vi "flash_RPCV2.vi"() -> ()   [LabVIEW 2017]
panel:
  out "error out 2":errorcluster
  out "Out 2":u8=4 format="%.0x"
  in  "Firmware":u16(ring)=4 items=["SP6"=4, "Middle"=3, "Final"=2]
  out "Out":u8 format="%.0x"
  out "字符串 2":string
  out "concatenated string":string
  in  "Register_Base_Address":u32=512 format="%x"
  in  "start":bool=TRUE
  out "Current IP address":string="192.168.10.20"
  in  "IP address list":string[](array[string])=["192.168.10.20"]
  in  "回读":bool
  out "Current Progress":u32(slide)=342016 scale=0.0..341712.0
  out "error out":errorcluster={"status"=TRUE, "code"=4, "source"="Read from Binary File in flash_RPCV1.vi<APPEND>\nG:\\rpc\\FPGA\\top.bin"}
  out "appended array":bool[](array[boolean])
  out "Process":u32=342016
  in  "error in (no error)":errorcluster
  in  "Read (TRUE)":bool
  out "byte data":string
  out "Total size (in bytes)":i64=341988
  in  "file path (use dialog)":path=path "G:/rpc/FPGA/top_sp6.bin"
  # "FF80 0001 0000 0209 13"
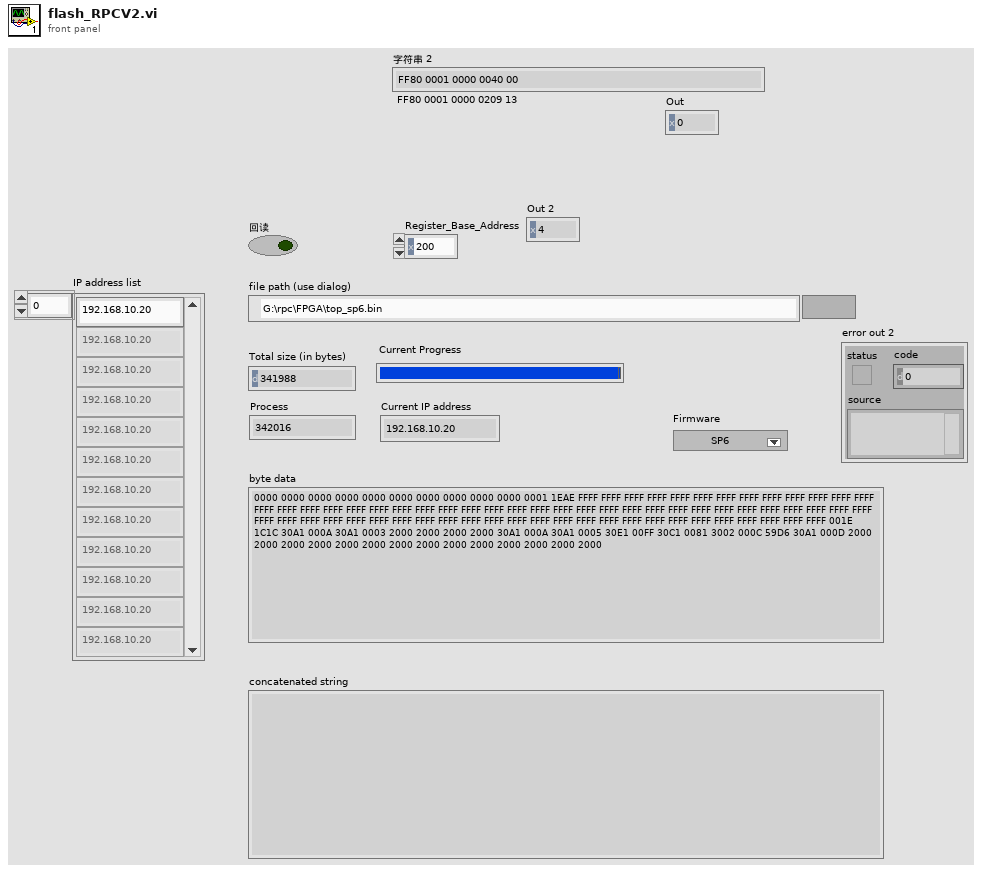
[diagram p1: front panel]
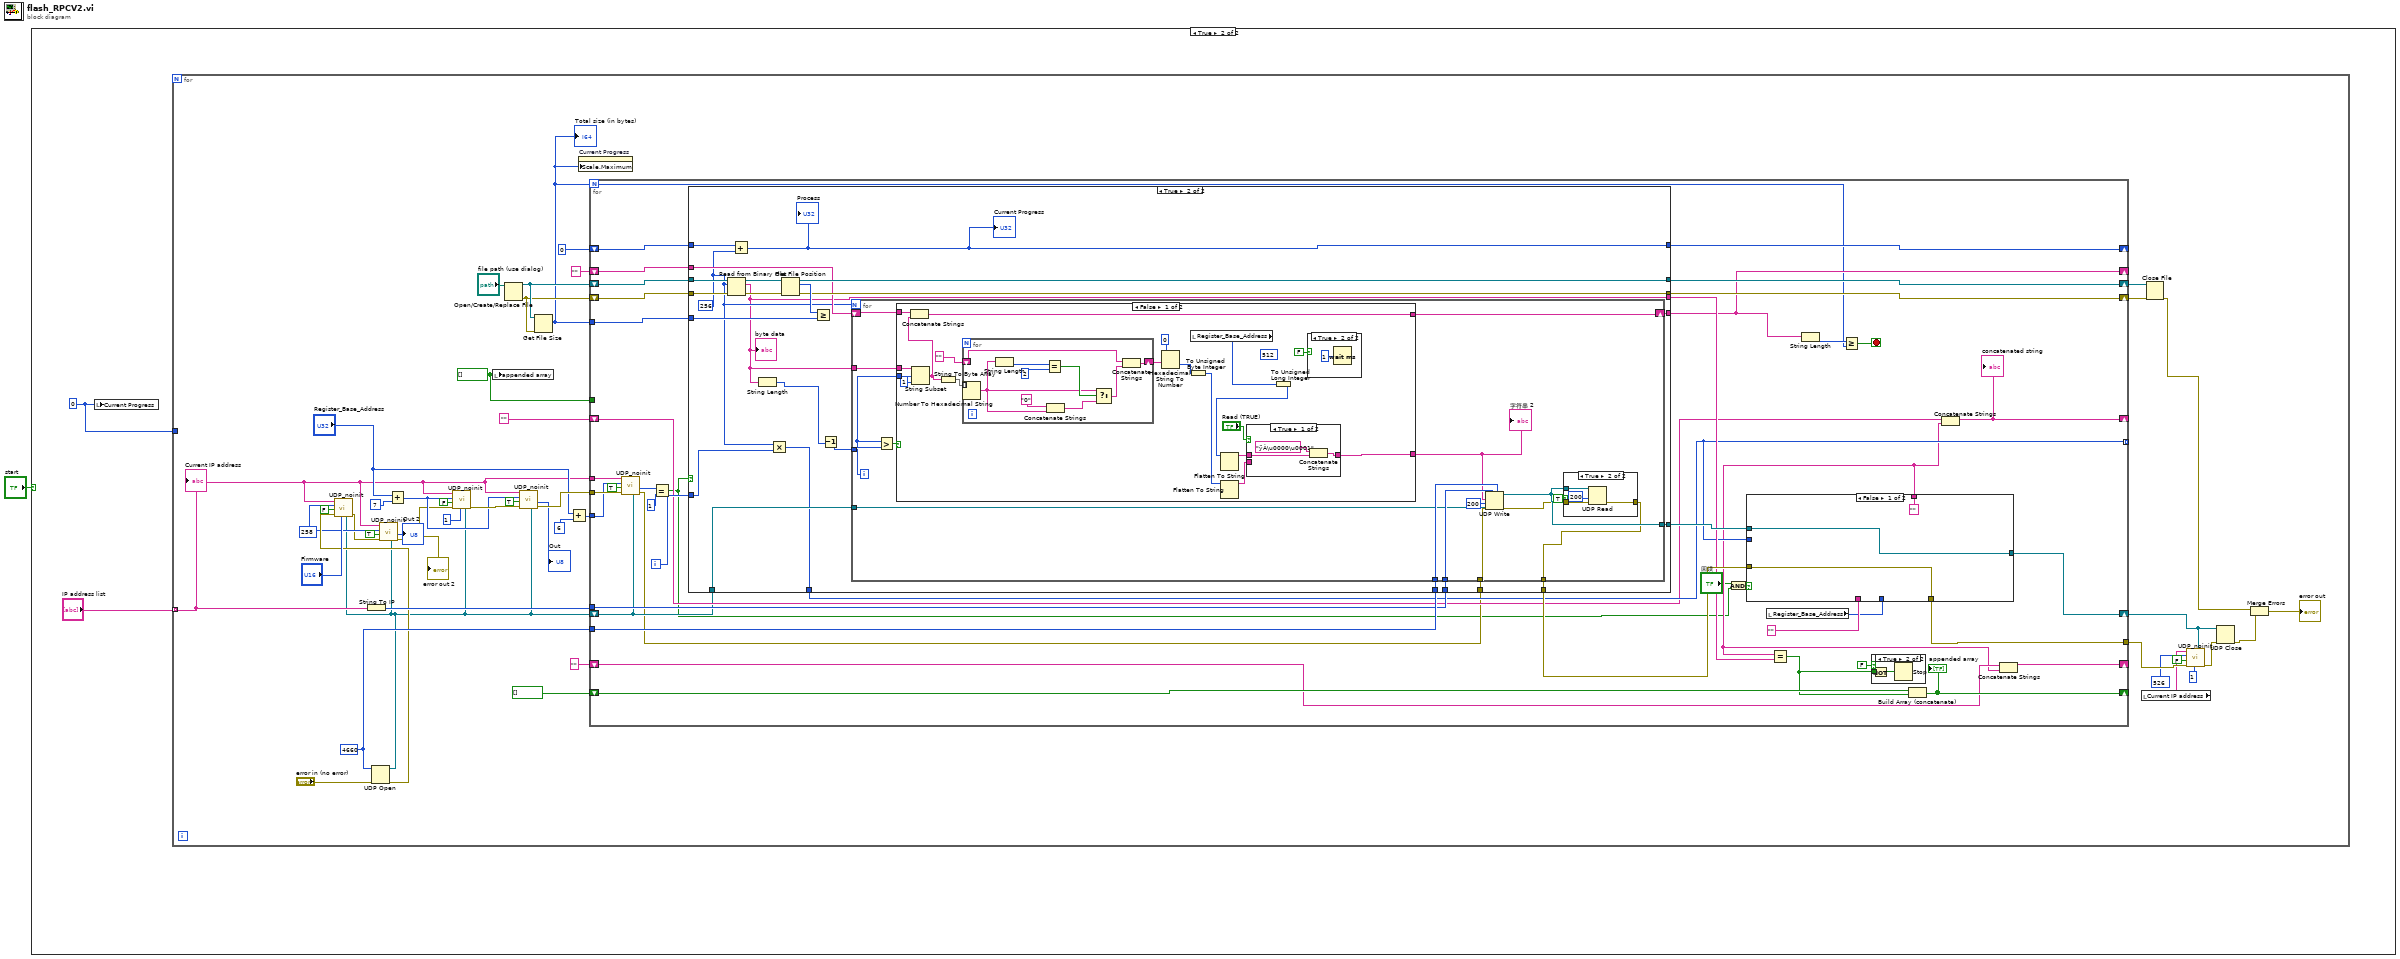
[diagram p0: block diagram]
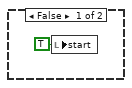
[diagram p2: hidden frame]
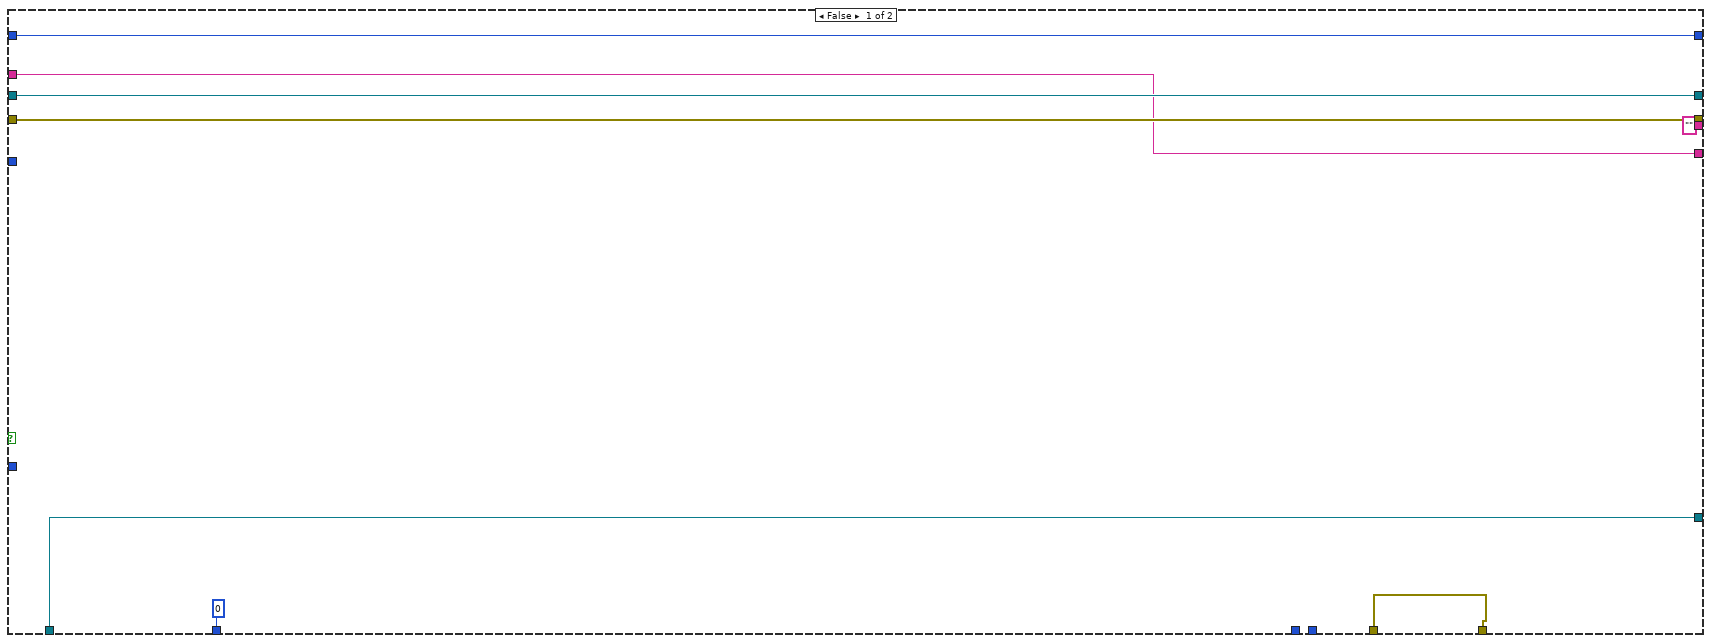
[diagram p3: hidden frame]
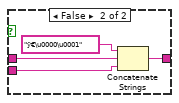
[diagram p5: hidden frame]
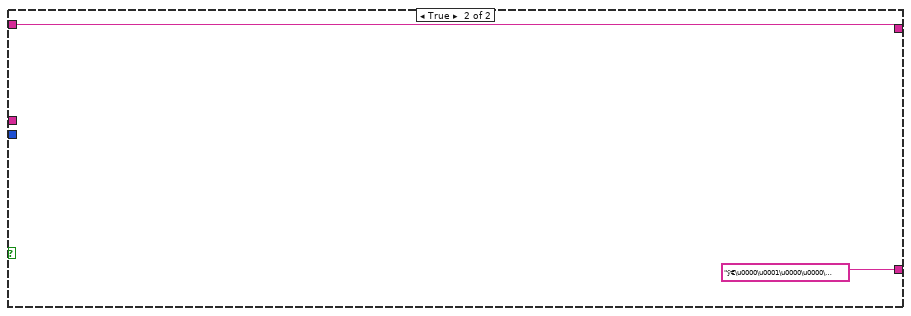
[diagram p7: hidden frame]
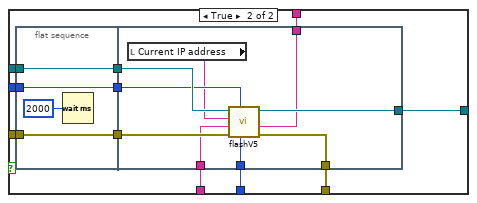
[diagram p8: hidden frame]
diagram:
  n1 = case shown="True" "start" {
    frame False {
      n2 = local write "start"(TRUE ("start")) -> ()
    }
    frame True {
      w3 = u8 0 ("In")
      n3 = local write "Current Progress"(w3) -> ()
      n4 = for {
        tunnel: "IP address list" -> [w18] mode=indexing
        tunnel: w3 -> [_]
        w17 = u32 258 ("Address")
        w32 = bool[] [] ("appended array")
        w45 = u16 4660 ("UDP port")
        n5 = String To IP(1:w18) -> (0:w44:u32)
        n6 = UDP Open(8:"error in (no error)", 11:w45) -> (port=w14:refnum<k16>, 0:w19:errorcluster)  [unwired: 3 in, 1 out]
        n7 = call "UDP_noinit.vi"("connection ID"=w14, "In"="Firmware", "error in (no error)"=w19, "Read (TRUE)"=FALSE, "Address"=w17, "IP address"=w18) -> ("error out"=w13:errorcluster)  [unwired: 2 in, 2 out]
        n8 = call "UDP_noinit.vi"("connection ID"=w14, "error in (no error)"=w13, "Read (TRUE)"=TRUE, "Address"=w17, "IP address"=w18) -> ("error out"=w12:errorcluster, "Out"=→"Out 2":u8)  [unwired: 3 in, 1 out]
        "error out 2" <- w12
        n9 = Add(x="Register_Base_Address", y=u32 7 ("Address")) -> (x+y=w27:u32)
        n10 = call "UDP_noinit.vi"("connection ID"=w14, "In"=u8 1, "error in (no error)"=w12, "Read (TRUE)"=FALSE, "Address"=w27, "IP address"=w18) -> ("error out"=w36:errorcluster)  [unwired: 2 in, 2 out]
        n11 = local write "appended array"(w32) -> ()
        n12 = Open/Create/Replace File(file path (use dialog)="file path (use dialog)") -> (refnum out=w49:refnum<file>, error out=w48:errorcluster)  [unwired: 5 in, 1 out]
        n13 = call "UDP_noinit.vi"("connection ID"=w14, "error in (no error)"=w36, "Read (TRUE)"=TRUE, "Address"=w27, "IP address"=w18) -> ("error out"=w38:errorcluster, "Out"=→"Out":u8)  [unwired: 3 in, 1 out]
        n14 = Get File Size(file=w49, error in=w48) -> (size (in bytes)=w33:i64)  [unwired: 2 out]
        "Total size (in bytes)" <- w33
        n15 = Add(x="Register_Base_Address", y=u32 6 ("Address")) -> (x+y=w24:u32)
        n16 = property on="Current Progress" class="Slide (strict)"("Scale.Maximum"=w33) -> ()  [unwired: 2 in, 2 out]
        n17 = for {
          N: w33 -> [w70]
          tunnel: w33 -> [w91]
          shift-right: [w90] -> w47
          shift-left: w48 -> [w92]
          shift-right: [w89] -> w46
          shift-left: w49 -> [w93]
          shift-right: [w72] -> _
          shift-left: "" -> [w88]
          tunnel: w45 -> [w85]
          tunnel: [w80] -> w10
          tunnel: w44 -> [w84]
          shift-right: [w82] -> w6
          shift-left: w14 -> [w60]
          shift-right: [w86] -> _
          shift-left: u32 0 ("length (rest)") -> [w87]
          shift-right: [w77] -> _
          shift-left: bool[] [] -> [w75]
          tunnel: [w73] -> _ mode=indexing
          shift-right: [w68] -> _
          shift-left: "" -> [w67]
          tunnel: w18 -> [w65]
          tunnel: w38 -> [w59]
          shift-right: [w57] -> _
          shift-left: "" -> [w56]
          tunnel: w32 -> [_]
          tunnel: w24 -> [w52]
          i -> [w78]
          stop <- w69 stop-if-true
          n18 = call "UDP_noinit.vi"("connection ID"=w60, "error in (no error)"=w59, "Read (TRUE)"=TRUE, "Address"=w52, "IP address"=w65) -> ("error out"=w58:errorcluster, "Out"=w63:u8)  [unwired: 3 in, 1 out]
          n19 = Equal?(x=w63, y=u8 1) -> (x = y?=w54:bool)
          n20 = case shown="True" w54 {
            tunnel: w93 -> [w98 w125]
            tunnel: w92 -> [w99 w124]
            tunnel: w91 -> [_ w120]
            tunnel: [w99 w119] -> w90
            tunnel: [w98 w118] -> w89
            tunnel: w88 -> [w96 w117]
            tunnel: w87 -> [w97 w116]
            tunnel: [w97 w102] -> w86
            tunnel: w85 -> [_ w115]
            tunnel: w84 -> [_ w114]
            tunnel: w58 -> [w100 w113]
            tunnel: w60 -> [w101 w112]
            tunnel: [w101 w109] -> w83
            tunnel: [w100 w108] -> w81
            tunnel: w78 -> [_ w107]
            tunnel: ["" w105] -> w76
            tunnel: [0 w104] -> w73
            tunnel: [w96 w103] -> w72
            frame False {
            }
            frame True {
              w106 = 256 ("count (1)")
              n21 = Read from Binary File(8:w124, 10:w106, 11:w125) -> (0:w122:errorcluster, 2:w105:string, 3:w123:refnum<file>)  [unwired: 3 in, 1 out]
              "byte data" <- w105
              n22 = Add(x=w116, y=w106) -> (x+y=w102:u32)
              "Process" <- w102
              "Current Progress" <- w102
              n23 = String Length(string=w105) -> (length=w111:i32)
              n24 = Multiply(x=w106, y=w107) -> (x*y=w104:i32)
              n25 = Get File Position(4:w122, 7:w123) -> (0:w119:errorcluster, 2:w121:i64, 3:w118:refnum<file>)
              n26 = Greater Or Equal?(x=w121, y=w120) -> ()  [unwired: 1 out]
              n27 = Decrement(x=w111) -> (x-1=w110:i32)
              n28 = for {
                N: w106 -> [_]
                tunnel: w105 -> [w141]
                shift-right: [w139] -> w103
                shift-left: w117 -> [w140]
                tunnel: w115 -> [w138]
                tunnel: w114 -> [w137]
                tunnel: w113 -> [w136]
                tunnel: w112 -> [w130]
                tunnel: [w126] -> w108
                tunnel: [w129] -> w109
                tunnel: w110 -> [w133]
                i -> [w132]
                n29 = Greater?(x=w132, y=w133) -> (0:w134:bool)
                n30 = case shown="False" w134 {
                  tunnel: w141 -> [w158 _]
                  tunnel: w140 -> [w156 w184]
                  tunnel: [w155 w184] -> w139
                  tunnel: w132 -> [w149 _]
                  tunnel: [w148 "ÿ€\u0000\u0001\u0000\u0000\u0000@\u0000" ("字符串 2")] -> w131
                  frame False {
                    (unwired) u32 512 ("Address")
                    n31 = String Subset(string=w158, offset (0)=w149, length (rest)=1 ("length (rest)")) -> (substring=w154:string)
                    n32 = Concatenate Strings(w156, w154) -> (w155:string)
                    n33 = String To Byte Array(string=w154) -> (unsigned byte array=w164:u8[])
                    n34 = for {
                      shift-right: [w182] -> w163
                      shift-left: "" ("format string") -> [w179]
                      tunnel: w164 -> [w183] mode=indexing
                      n35 = Number To Hexadecimal String(2:w183) -> (0:w175:string)  [unwired: 1 in]
                      n36 = String Length(string=w175) -> (length=w181:i32)
                      n37 = Equal?(x=w181, y=2) -> (x = y?=w178:bool)
                      n38 = Concatenate Strings("0" ("format string"), w175) -> (w177:string)
                      n39 = Select(t=w175, s=w178, f=w177) -> (s? t:f=w174:string)
                      n40 = Concatenate Strings(w179, w174) -> (w182:string)
                    }
                    n41 = Hexadecimal String To Number(string=w163, default (0uL)=u64 0 ("default (0 U32)")) -> (number=w161:u64)  [unwired: 1 in, 1 out]
                    n42 = To Unsigned Byte Integer(number=w161) -> (unsigned 8bit integer=w160:u8)
                    n43 = local read "Register_Base_Address"() -> (w147:u32)
                    n44 = Flatten To String(anything=w160) -> (data string=w151:string)  [unwired: 3 in, 2 out]
                    n45 = To Unsigned Long Integer(number=w147) -> (unsigned 32bit integer=w159:u32)
                    n46 = Flatten To String(anything=w159) -> (data string=w152:string)  [unwired: 3 in, 2 out]
                    n47 = case shown="True" "Read (TRUE)" {
                      tunnel: [w167 w171] -> w148
                      tunnel: w152 -> [w166 w170]
                      tunnel: w151 -> [_ w169]
                      frame True {
                        n48 = Concatenate Strings("ÿÀ\u0000\u0001" ("initial string"), w166) -> (w167:string)
                      }
                      frame False {
                        n49 = Concatenate Strings("ÿ€\u0000\u0001" ("initial string"), w170, w169) -> (w171:string)
                      }
                    }
                    n50 = case shown="True" FALSE {
                      frame False {
                      }
                      frame True {
                        n51 = Wait (ms)(milliseconds to wait=u32 1) -> ()  [unwired: 1 out]
                      }
                    }
                  }
                  frame True {
                  }
                }
                "字符串 2" <- w131
                n52 = UDP Write(address=w137, port or service name=w138, connection ID=w130, data in=w131, 8:w136, 9:200 ("timeout ms (25000)")) -> (error out=w127:errorcluster, 3:w129:refnum<k16>)
                n53 = case shown="True" TRUE {
                  tunnel: w129 -> [_ w146]
                  tunnel: w127 -> [w142 w145]
                  tunnel: [w142 w144] -> w126
                  frame False {
                  }
                  frame True {
                    n54 = UDP Read(connection ID=w146, timeout ms (25000)=200, 8:w145) -> (error out=w144:errorcluster)  [unwired: 5 out]
                  }
                }
              }
            }
          }
          n55 = And(x="回读", y=w54) -> (x .and. y?=w61:bool)
          n56 = local read "Register_Base_Address"() -> (w51:u32)
          n57 = case shown="False" w61 {
            tunnel: w83 -> [w188 w196]
            tunnel: [w188 w195] -> w82
            tunnel: w81 -> [w187 w194]
            tunnel: [w187 w193] -> w80
            tunnel: "" ("empty") -> [_ w192]
            tunnel: w73 -> [_ w191]
            tunnel: ["" ("String") w190] -> w55
            tunnel: w51 -> [_ w189]
            frame False {
            }
            frame True {
              n58 = flat-sequence {
                tunnel: w191 -> [w201]
                tunnel: w194 -> [w202]
                tunnel: w196 -> [w203]
                tunnel: [w203] -> w199
                tunnel: [w202] -> w198
                tunnel: [w201] -> w197
                tunnel: [w209] -> w193
                tunnel: w192 -> [w208]
                tunnel: [w207] -> w190
                tunnel: w199 -> [w212]
                tunnel: w198 -> [w210]
                tunnel: w197 -> [w206]
                tunnel: [w211] -> w195
                tunnel: w189 -> [w204]
                frame #0 {
                  n59 = Wait (ms)(milliseconds to wait=u32 2000) -> ()  [unwired: 1 out]
                }
                frame #1 {
                  n60 = local read "Current IP address"() -> (w205:string)
                  n61 = call "flashV5.vi"("Register_Base_Address"=w204, "flash_base_address"=w206, "error in (no error)"=w210, "empty"=w208, "address"=w205, "connection ID"=w212) -> ("error out"=w209:errorcluster, "String"=w207:string, "connection ID 2"=w211:refnum<k16>)  [unwired: 2 in, 1 out]
                }
              }
            }
          }
          n62 = Equal?(x=w55, y=w76) -> (x = y?=w74:bool)
          n63 = String Length(string=w72) -> (length=w71:i32)
          n64 = Greater Or Equal?(x=w71, y=w70) -> (x >= y?=w69:bool)
          n65 = case shown="True" FALSE {
            tunnel: w74 -> [_ w213]
            frame False {
            }
            frame True {
              n66 = Not(x=w213) -> (.not. x?=w214:bool)
              n67 = Stop(stop? (T)=w214) -> ()
            }
          }
          n68 = Build Array (concatenate)(w75, w74) -> (w77:bool[])
          "appended array" <- w77
          n69 = Concatenate Strings(w67, w55) -> (w68:string)
          "concatenated string" <- w68
          n70 = Concatenate Strings(w56, w55) -> (w57:string)
        }
        n71 = local read "Current IP address"() -> (w8:string)
        n72 = Close File(refnum=w46, error in=w47) -> (error out=w31:errorcluster)  [unwired: 1 out]
        n73 = call "UDP_noinit.vi"("connection ID"=w6, "In"=u8 1, "error in (no error)"=w10, "Read (TRUE)"=FALSE, "Address"=u32 526, "IP address"=w8) -> ("error out"=w7:errorcluster)  [unwired: 2 in, 2 out]
        n74 = UDP Close(connection ID=w6, 8:w7) -> (error out=w30:errorcluster)  [unwired: 1 out]
        n75 = Merge Errors(w31, w30) -> (→"error out":errorcluster)
        "Current IP address" <- w18
      }
    }
  }
